vi "配置和范例.vi"() -> ()   [LabVIEW 2010]
uses:
  <vilib>/DAQmx/read.llb/DAQmx Read (Analog 1D Wfm NChan NSamp).vi
  <vilib>/daqmx/miscellaneous.llb/DAQmx Fill In Error Info.vi
panel:
  out "task out":refnum<k21>
  out "data 3":waveform(dbl)[](graph) caption="data"
  in  "stop 2":bool caption="stop"
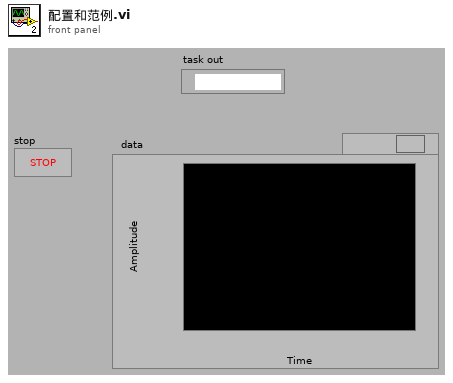
[diagram p1: front panel]
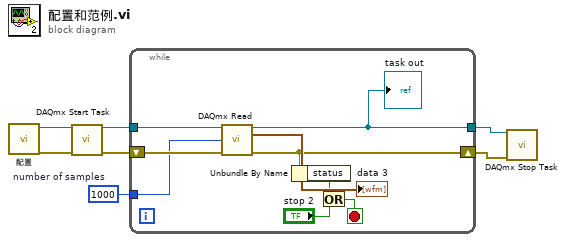
[diagram p0: block diagram]
diagram:
  w5 = 1000  # number of samples
  n1 = call "配置.vi"() -> ("error out"=w1:errorcluster, "task out"=w2:refnum<k21>)  [unwired: 10 in]
  n2 = call <vilib>:"DAQmx Start Task.vi"("task/channels in"=w2, "error in"=w1) -> ("task out"=w7:refnum<k21>, "error out"=w6:errorcluster)  [unwired: 12 in]
  n3 = while "While循环" {
    tunnel: w7 -> [w16]
    tunnel: w5 -> [w12]
    tunnel: [w13] -> w3
    shift-right: [w10] -> w4
    shift-left: w6 -> [w15]
    stop <- w9 stop-if-true
    n4 = call-poly <vilib>:"DAQmx Read.vi"("task/channels in"=w16, "number of samples per channel"=w12, "error in"=w15) -> ("task out"=w13:refnum<k21>, "data"=→"data 3":waveform(dbl)[], "error out"=w10:errorcluster)  [unwired: 10 in]
    "task out" <- w13
    n5 = Unbundle By Name(w10) -> ("status"=w11:bool)
    n6 = Or(x=w11, y="stop 2") -> (x .or. y?=w9:bool)
  }
  n7 = call <vilib>:"DAQmx Stop Task.vi"("task/channels in"=w3, "error in"=w4) -> ()  [unwired: 12 in, 2 out]
